vi "TIO Access Module Init.vi"(9 "ID":string="Twinleaf", 11 "URL":refnum<visa-resource-name>="tcp://localhost") -> (0 "error out":errorcluster={"status"=TRUE, "code"=-1073807252, "source"="VISA Read in SLIP Decode Serial Read.vi->NN VISA Read.vi->NN RPC.vi"}, 1 "Connected":bool, 3 "TS Connection":T1={"Type"=enum."TCP", "Serial"="serial:///dev/cu.usbserial-00000", "TCP"=refnum, "Timeout"=500})   [LabVIEW 2017]
uses:
  <instrlib>/tio-labview/TIO Library/Socket/Helpers/TIO Serial Port Name Search.vi
  <instrlib>/tio-labview/TIO Library/RPC/TIO RPC Blocking.vi
  <vilib>/Utility/error.llb/Clear Errors.vi
  <instrlib>/tio-labview/TIO Library/RPC/TIO RPC Send REQuest.vi
  <instrlib>/tio-labview/TIO Library/Socket/TIO Stream Read.vi
  <instrlib>/tio-labview/TIO Library/RPC/RPC Helpers/TIO RPC Parse Reply.vi
  <instrlib>/tio-labview/TIO Library/Socket/TIO Stream Write.vi
  <instrlib>/tio-labview/TIO Library/RPC/RPC Helpers/TIO RPC Form Request.vi
  <instrlib>/tio-labview/TIO Library/Socket/Helpers/TIO Parse Packet.vi
  <instrlib>/tio-labview/TIO Library/Socket/Helpers/TIO SLIP Serial Read.vi
  <instrlib>/tio-labview/TIO Library/Socket/Helpers/TIO SLIP Serial Write.vi
  <instrlib>/tio-labview/TIO Library/Socket/Helpers/TIO Form Packet.vi
  <instrlib>/tio-labview/TIO Library/Socket/Helpers/TIO Serial Checksum CRC32.vi
  <instrlib>/tio-labview/TIO Library/Socket/Helpers/TIO SLIP Encode.vi
  <vilib>/Instr/_visa.llb/VISA Configure Serial Port (Instr).vi
  <instrlib>/tio-labview/TIO Library/Socket/Helpers/TIO Serial Port Discovery.vi
panel:
  out "ID Verified":string
  out "ID Verified":bool
  # "TIO Proxy Init"
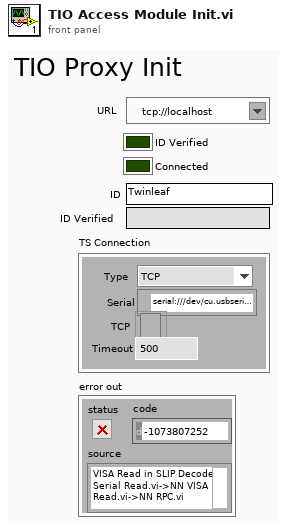
[diagram p1: front panel]
types:
  T1 = cluster{"Type":enum16{"TCP", "Serial"}, "Serial":refnum<visa-resource-name>, "TCP":refnum<k5>, "Timeout":u32}
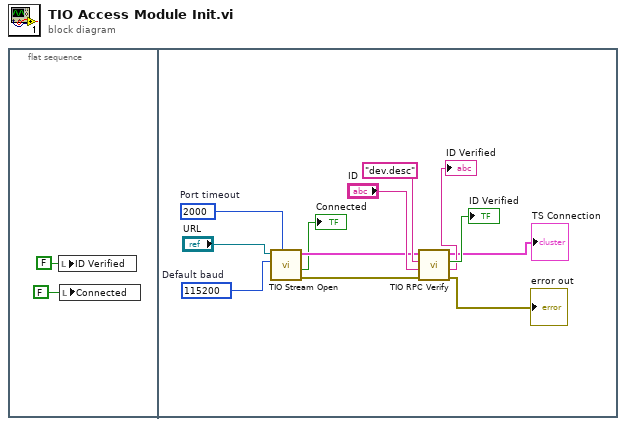
[diagram p0: block diagram]
diagram:
  n1 = flat-sequence {
    frame #0 {
      n2 = local write "ID Verified"(FALSE ("ID 2")) -> ()
      n3 = local write "Connected"(FALSE ("Quit")) -> ()
    }
    frame #1 {
      w12 = u32 115200  # Default baud
      w11 = u32 2000  # Port timeout
      n4 = call <instrlib>:"TIO Stream Open.vi"("Port timeout"=w11, "Default baud"=w12, "URL"="URL") -> ("error out"=w6:errorcluster, "Connected"=→"Connected":bool, "TS Connection"=w10:T1)  [unwired: 6 in]
      n5 = call <instrlib>:"TIO RPC Verify.vi"("error in (no error)"=w6, "Starts With"="ID", "Topic"="dev.desc", "TS Connection"=w10) -> ("error out"=→"error out":errorcluster, "Respose"=→"ID Verified":string, "Verify"=→"ID Verified":bool, "TS Connection"=→"TS Connection":T1)  [unwired: 4 in]
    }
  }
